vi "_readObject.vi"(8 "error in (no error)":errorcluster, 11 "JSONParser in":refnum<class "tJSONParser.lvclass">) -> (0 "error out":errorcluster, 2 "tBSONDocument out":refnum<class "tBSONDocument.lvclass">, 3 "JSONParser out":refnum<class "tJSONParser.lvclass">)   [LabVIEW 2013, in "JSON.lvlib" / "tJSONParser.lvclass"]
doc: "Read JSON object enclosed by {} into a tBSONDocument object. Errors are returned if a string value pair isn't found after the '{' and after every comma."
uses:
  tJSONParser.lvclass
  BSON/tBSONDocument/tBSONDocument.lvclass
  tJSONParser.lvclass/tJSONParser.ctl
  _error.ctl
  _tokenType.ctl
  BSON/tBSONElement/setName.vi
  BSON/tBSONElement/tBSONElement.lvclass
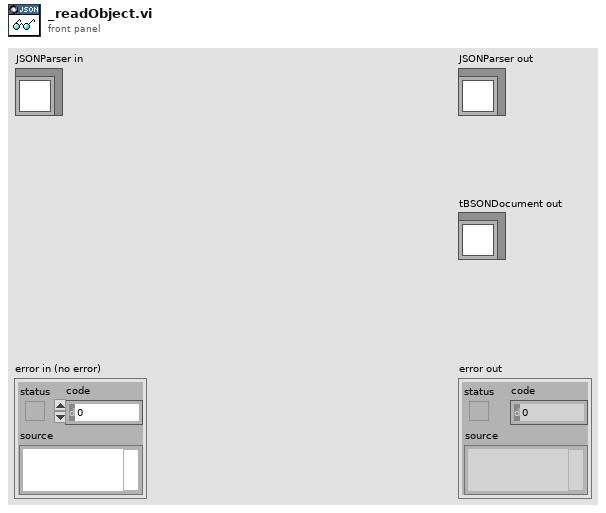
[diagram p1: front panel]
types:
  T1 = typedef "JSON.lvlib/tJSONParser.lvclass/_tokenType.ctl" = enum16{"Object Begin", "Object End", "Array Begin", "Array End", "String Delimeter", "Forward Slash", "Number", "Boolean", "Null", "Object Or Array Separator", "Pair Separator", "End Of File", "Asterisk", "Backward Slash", "Other"}
  T2 = typedef "JSON.lvlib/tJSONParser.lvclass/_error.ctl" = enum16{"Missing Object Open", "Missing Pair Separator", "Missing Object End Or Separator", "Missing Pair String", "Unexpected Token", "Missing Array End Or Separator", "Invalid Escape Sequence", "Unexpected End Of File", "Invalid Unicode", "Unexpected End Of Line", "Invalid Numerical Constant"}
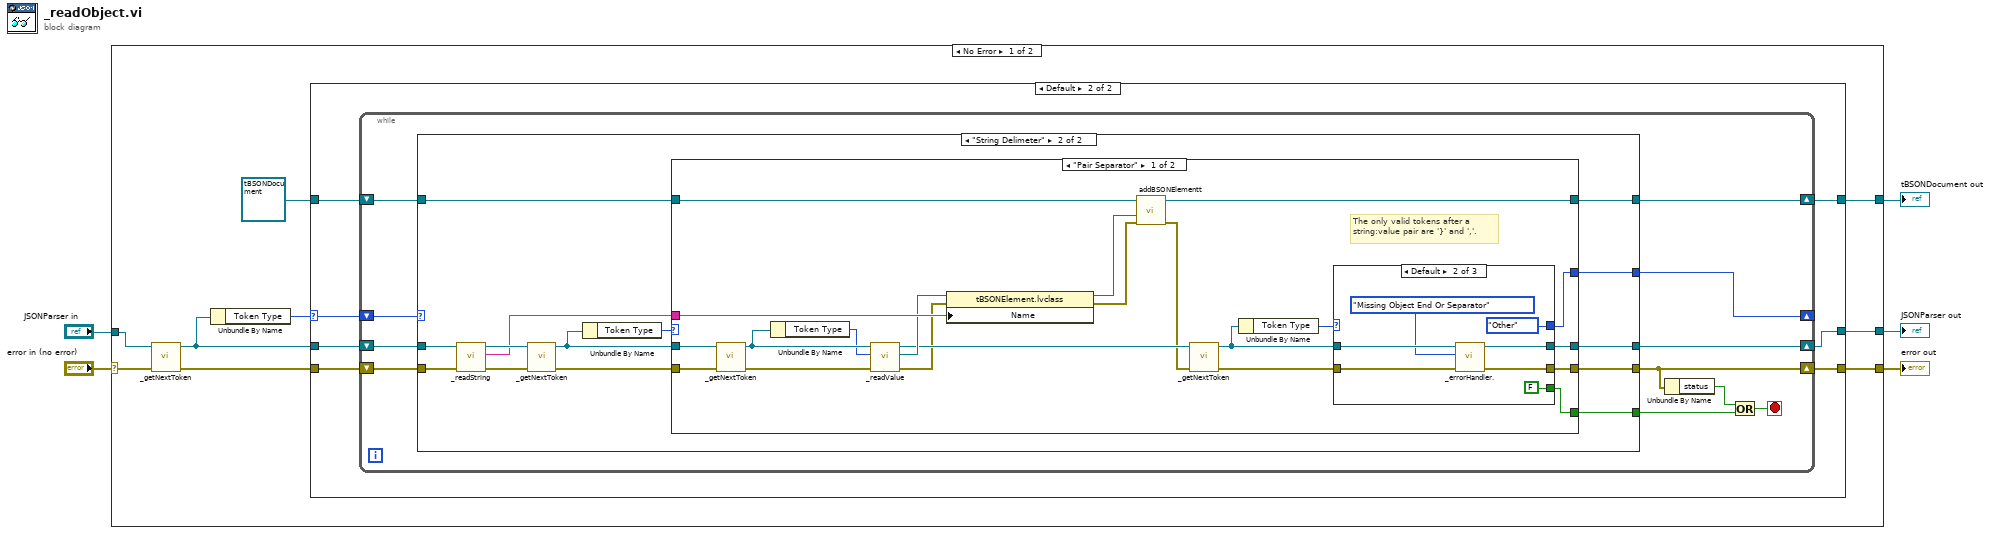
[diagram p0: block diagram]
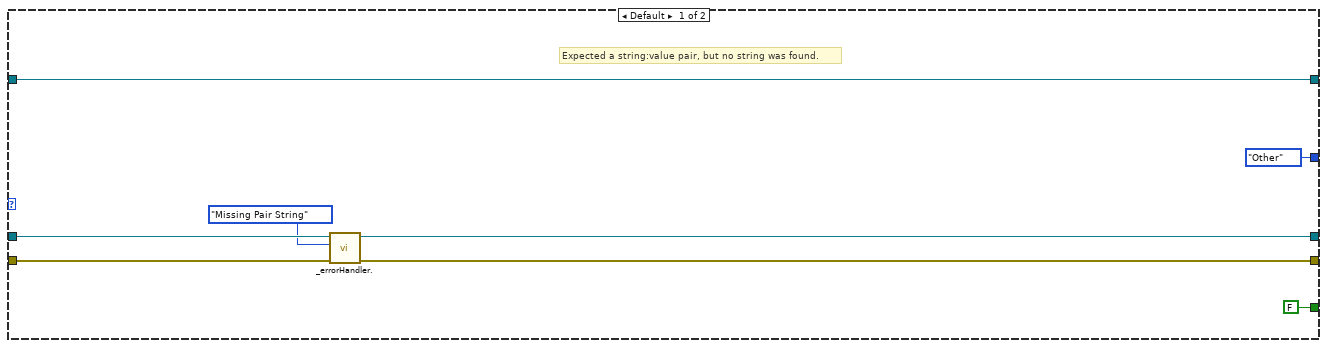
[diagram p3: hidden frame]
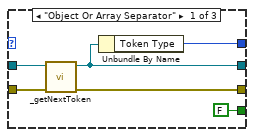
[diagram p4: hidden frame]
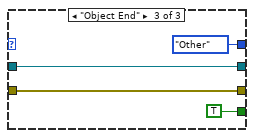
[diagram p5: hidden frame]
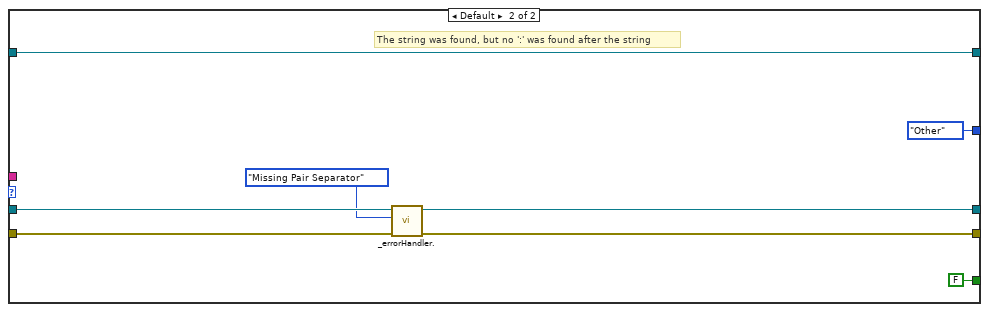
[diagram p6: hidden frame]
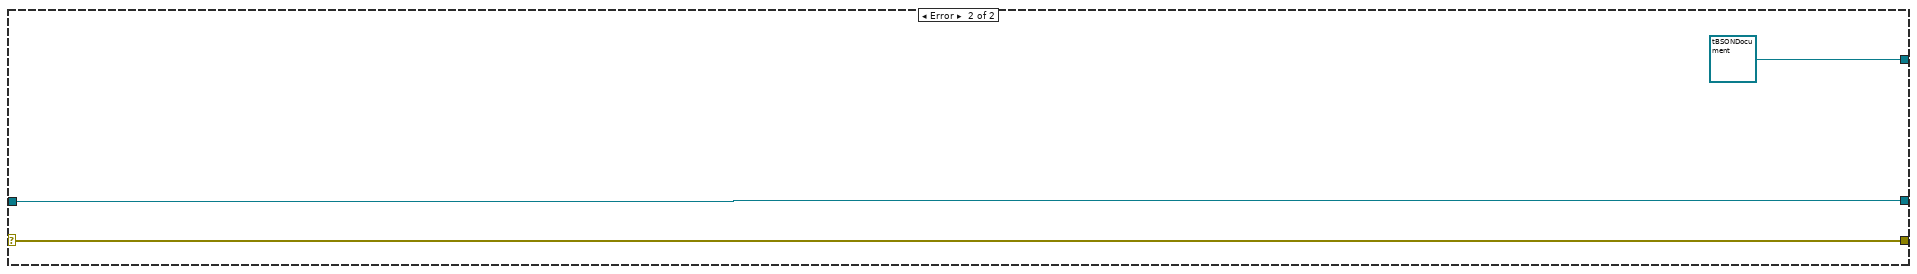
[diagram p7: hidden frame]
diagram:
  n1 = case shown="No Error" "error in (no error)" {
    selector: "error in (no error)" -> [w11 w106]
    tunnel: [w14 w106] -> w4
    tunnel: [w13 w105] -> w2
    tunnel: "JSONParser in" -> [w10 w105]
    tunnel: [w12 refnum<class "tBSONDocument.lvclass"> refnum ("lvMongoDriver.lvlib:BSON.lvlib:tBSONDocument.lvclass")] -> w1
    frame No Error {
      n2 = call "_getNextToken.vi"("error in (no error)"=w11, "JSON Parser In"=w10) -> ("error out"=w9:errorcluster, "JSON Parser Out"=w8:refnum<class "tJSONParser.lvclass">)  [unwired: 8 in]
      n3 = Unbundle By Name(w8) -> ("Token Type"=w7:T1)
      n4 = case shown="Default" w7 {
        selector: w7 -> [_ w18]
        tunnel: [w16 w24] -> w14
        tunnel: [w17 w23] -> w13
        tunnel: [w15 w22] -> w12
        tunnel: w9 -> [w16 w19]
        tunnel: w8 -> [w17 w20]
        tunnel: refnum<class "tBSONDocument.lvclass"> refnum ("tBSONDocument out") -> [w15 w21]
        frame "Object End" {
          # "Empty Object"
        }
        frame Default {
          n5 = while {
            shift-right: [w29] -> w24
            shift-left: w19 -> [w27]
            shift-right: [w35] -> w23
            shift-left: w20 -> [w28]
            shift-right: [w30] -> w22
            shift-left: w21 -> [w31]
            shift-right: [w25] -> _
            shift-left: w18 -> [w26]
            stop <- w33 stop-if-true
            n6 = case shown="\"String Delimeter\"" w26 {
              tunnel: w27 -> [w41 w54]
              tunnel: [w40 w56] -> w29
              tunnel: w28 -> [w43 w53]
              tunnel: [w42 w55] -> w35
              tunnel: [FALSE w45] -> w32
              tunnel: w31 -> [w37 w46]
              tunnel: [w37 w47] -> w30
              tunnel: [_tokenType."Other" ("Token Type") w44] -> w25
              frame Default {
                # "Expected a string:value pair, but no string was found."
                n7 = call "_errorHandler..vi"("error in (no error)"=w41, "Error Type"=_error."Missing Pair String", "JSON Parser In"=w43) -> ("error out"=w40:errorcluster, "JSON Parser Out"=w42:refnum<class "tJSONParser.lvclass">)  [unwired: 7 in]
              }
              frame "String Delimeter" {
                n8 = call "_readString.vi"("error in (no error)"=w54, "JSONParser in"=w53) -> ("error out"=w51:errorcluster, "String"=w50:string, "JSONParser out"=w52:refnum<class "tJSONParser.lvclass">)  [unwired: 7 in]
                n9 = call "_getNextToken.vi"("error in (no error)"=w51, "JSON Parser In"=w52) -> ("error out"=w57:errorcluster, "JSON Parser Out"=w49:refnum<class "tJSONParser.lvclass">)  [unwired: 8 in]
                n10 = Unbundle By Name(w49) -> ("Token Type"=w48:T1)
                n11 = case shown="\"Pair Separator\"" w48 {
                  tunnel: w57 -> [w70 w103]
                  tunnel: [w60 w102] -> w56
                  tunnel: [w61 w101] -> w55
                  tunnel: w49 -> [w69 w100]
                  tunnel: w50 -> [w78 _]
                  tunnel: [w76 w98] -> w47
                  tunnel: w46 -> [w75 w98]
                  tunnel: [w62 FALSE] -> w45
                  tunnel: [w58 _tokenType."Other" ("Token Type")] -> w44
                  frame "Pair Separator" {
                    # "The only valid tokens after a\nstring:value pair are '}' and ','."
                    n12 = call "_getNextToken.vi"("error in (no error)"=w70, "JSON Parser In"=w69) -> ("error out"=w68:errorcluster, "JSON Parser Out"=w67:refnum<class "tJSONParser.lvclass">)  [unwired: 8 in]
                    n13 = Unbundle By Name(w67) -> ("Token Type"=w66:T1)
                    n14 = call "_readValue.vi"("error in (no error)"=w68, "Token Type"=w66, "JSONParser in"=w67) -> ("error out"=w71:errorcluster, "tBSONElement Out"=w77:refnum<class "tBSONElement.lvclass">, "JSONParser out"=w72:refnum<class "tJSONParser.lvclass">)  [unwired: 6 in]
                    n15 = property class="tBSONElement.lvclass"(reference=w77, error in=w71, "Name"=w78) -> (reference out=w74:refnum<class "tBSONElement.lvclass">, error out=w73:errorcluster)
                    n16 = call "addBSONElementt.vi"("error in (no error)"=w73, "Element"=w74, "tBSONDocument in"=w75) -> ("error out"=w65:errorcluster, "tBSONDocument out"=w76:refnum<class "tBSONDocument.lvclass">)  [unwired: 7 in]
                    n17 = call "_getNextToken.vi"("error in (no error)"=w65, "JSON Parser In"=w72) -> ("error out"=w64:errorcluster, "JSON Parser Out"=w63:refnum<class "tJSONParser.lvclass">)  [unwired: 8 in]
                    n18 = Unbundle By Name(w63) -> ("Token Type"=w59:T1)
                    n19 = case shown="Default" w59 {
                      tunnel: w64 -> [w83 w90 w94]
                      tunnel: w63 -> [w82 w89 w93]
                      tunnel: [FALSE FALSE TRUE] -> w62
                      tunnel: [w81 w87 w94] -> w60
                      tunnel: [w80 w88 w93] -> w61
                      tunnel: [w79 _tokenType."Other" ("Token Type") _tokenType."Other" ("Token Type")] -> w58
                      frame "Object Or Array Separator" {
                        n20 = call "_getNextToken.vi"("error in (no error)"=w83, "JSON Parser In"=w82) -> ("error out"=w81:errorcluster, "JSON Parser Out"=w80:refnum<class "tJSONParser.lvclass">)  [unwired: 8 in]
                        n21 = Unbundle By Name(w80) -> ("Token Type"=w79:T1)
                      }
                      frame Default {
                        n22 = call "_errorHandler..vi"("error in (no error)"=w90, "Error Type"=_error."Missing Object End Or Separator", "JSON Parser In"=w89) -> ("error out"=w87:errorcluster, "JSON Parser Out"=w88:refnum<class "tJSONParser.lvclass">)  [unwired: 7 in]
                      }
                      frame "Object End" {
                      }
                    }
                  }
                  frame Default {
                    # "The string was found, but no ':' was found after the string"
                    n23 = call "_errorHandler..vi"("error in (no error)"=w103, "Error Type"=_error."Missing Pair Separator", "JSON Parser In"=w100) -> ("error out"=w102:errorcluster, "JSON Parser Out"=w101:refnum<class "tJSONParser.lvclass">)  [unwired: 7 in]
                  }
                }
              }
            }
            n24 = Unbundle By Name(w29) -> ("status"=w34:bool)
            n25 = Or(x=w34, y=w32) -> (x .or. y?=w33:bool)
          }
        }
      }
    }
    frame Error {
    }
  }
  "error out" <- w4
  "JSONParser out" <- w2
  "tBSONDocument out" <- w1
